vi "Draw Polygon (SubVI).vi"(8 "color)":u32(colorbox)=65337, 9 "New Point":cluster{"X":dbl, "Y":dbl}, 10 "Nbr Polygon Points":i32=4, 11 "Selection Mask in":T1) -> (2 "new picture":picture, 3 "Selection Mask out":T1 {"Polygon"."Y [px]" format="%#_5g"; "Polygon"."X [px]" format="%#_5g"})   [LabVIEW 2023, in "Camera Calibration.lvlib"]
uses:
  Camera Calibration.lvlib
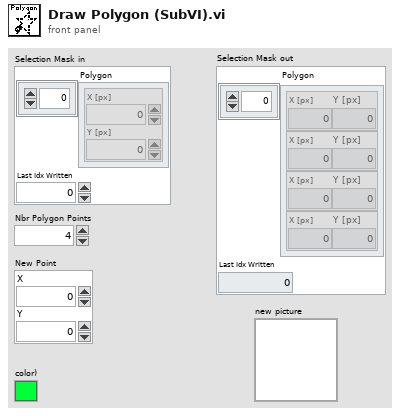
[diagram p1: front panel]
types:
  T1 = cluster{"Polygon":cluster{"X [px]":dbl, "Y [px]":dbl}[], "Last Idx Written":i32}
  T2 = cluster{"Width":u16, "Style":enum32{"Solid", "Dash", "Dot", "DashDot", "DashDotDot"}}
  T3 = cluster{"Polygon":cluster{"X [px]":dbl, "Y [px]":dbl}[], "lower limit":i32}
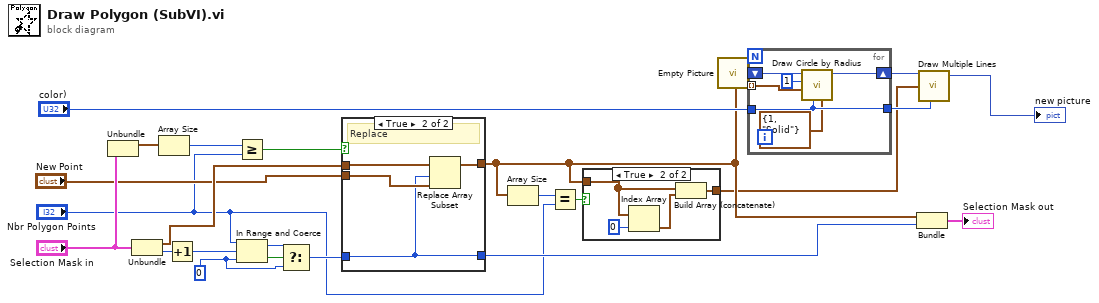
[diagram p0: block diagram]
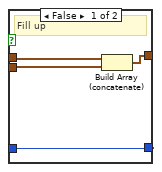
[diagram p3: hidden frame]
diagram:
  w11 = 0 ("lower limit")
  n1 = Unbundle("Selection Mask in") -> ("Polygon"=w20:cluster{"X [px]":dbl, "Y [px]":dbl}[])  [unwired: 1 out]
  n2 = Unbundle("Selection Mask in") -> ("Polygon"=w17:cluster{"X [px]":dbl, "Y [px]":dbl}[], "Last Idx Written"=w22:i32)
  n3 = Array Size(array=w20) -> (size(s)=w19:i32)
  n4 = Increment(x=w22) -> (x+1=w23:i32)
  n5 = Greater Or Equal?(x=w19, y="Nbr Polygon Points") -> (x >= y?=w18:bool)
  n6 = In Range and Coerce(upper limit="Nbr Polygon Points", x=w23, lower limit=w11) -> (coerced(x)=w12:i32, In Range?=w14:bool)
  n7 = Select(t=w12, s=w14, f=w11) -> (s? t:f=w13:i32)
  n8 = case shown="True" w18 {
    tunnel: w13 -> [w26 w29]
    tunnel: w17 -> [w28 w31]
    tunnel: "New Point" -> [w27 w32]
    tunnel: [w26 w29] -> w6
    tunnel: [w25 w30] -> w3
    frame False {
      # "Fill up"
      n9 = Build Array (concatenate)(w28, w27) -> (w25:cluster{"X":dbl, "Y":dbl}[])
    }
    frame True {
      # "Replace"
      n10 = Replace Array Subset(array=w31, new element=w32, index=w29) -> (w30:cluster{"X [px]":dbl, "Y [px]":dbl}[])
    }
  }
  n11 = Array Size(array=w3) -> (size(s)=w4:i32)
  n12 = Equal?(x=w4, y="Nbr Polygon Points") -> (x = y?=w5:bool)
  n13 = case shown="True" w5 {
    tunnel: w3 -> [w33 w35]
    tunnel: [w33 w34] -> w2
    frame False {
    }
    frame True {
      n14 = Index Array(array=w35, index=0) -> (element=w37:cluster{"X [px]":dbl, "Y [px]":dbl})
      n15 = Build Array (concatenate)(w35, w37) -> (w34:cluster{"X [px]":dbl, "Y [px]":dbl}[])
    }
  }
  n16 = call "Empty Picture"() -> ("empty picture"=w7:picture)
  n17 = for {
    tunnel: w3 -> [w43] mode=indexing
    shift-right: [w42] -> w10
    shift-left: w7 -> [w39]
    tunnel: "color)" -> [w41]
    tunnel: [w41] -> w8
    n18 = call <vilib>:"Draw Circle by Radius.vi"("pen"=T2 {"Width"=1, "Style"=enum."Solid"}, "color(black)"=w41, "pixel center"=w43, "radius"=i16 1, "picture"=w39) -> ("new picture"=w42:picture)  [unwired: 6 in]
  }
  n19 = Bundle("Polygon"=w3, "lower limit"=w6) -> (→"Selection Mask out":T3)  [unwired: 1 in]
  n20 = call <vilib>:"Draw Multiple Lines.vi"("picture"=w10, "line endpoints"=w2, "color(black)"=w8) -> ("new picture"=→"new picture":picture)  [unwired: 6 in]
